vi "PM100D_Initialize.vi"() -> (4 "VISA out":refnum<visa-resource-name>, 6 "Ranges":string[](array[string]), 8 "Instrument":string, 10 "Connected":bool, 15 "error out":errorcluster)   [LabVIEW 2015]
doc: "This VI scans for connected devices, that can be selected in a dialog box. Next steps\n- setting timeout\n- performing identification query\n- configuring the operation register to '512'; flag gets to HI when a new measurement value is ready to fetch\n- clear operation register"
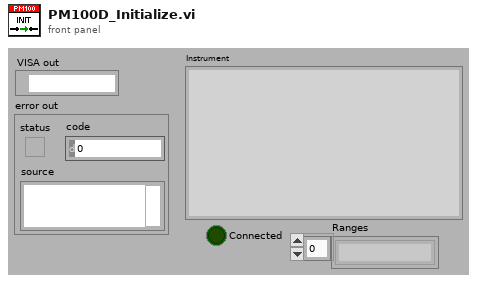
[diagram p1: front panel]
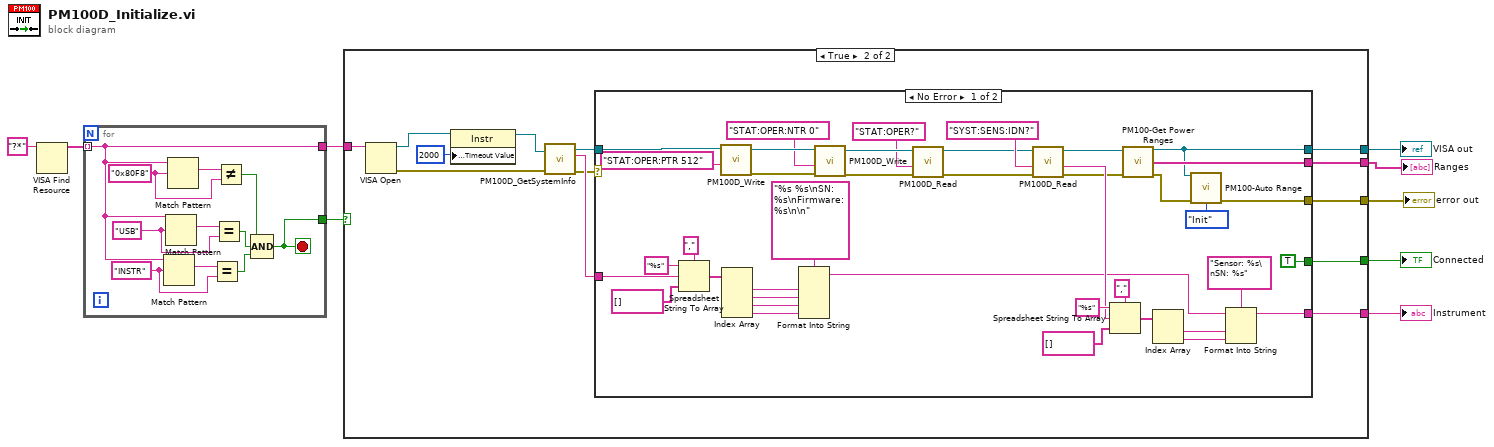
[diagram p0: block diagram]
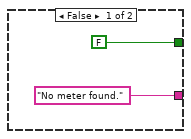
[diagram p2: hidden frame]
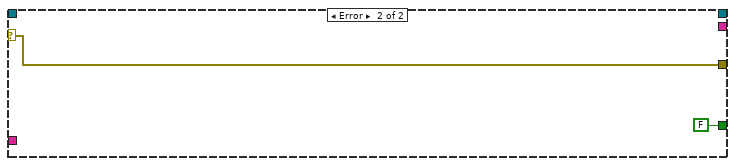
[diagram p3: hidden frame]
diagram:
  n1 = VISA Find Resource(11:"?*" ("expression (\"?*\")")) -> (3:w6:string[])  [unwired: 1 in, 3 out]
  n2 = for {
    tunnel: w6 -> [w11] mode=indexing
    tunnel: [w11] -> w5
    tunnel: [w10] -> w4
    stop <- w10 stop-if-true
    w12 = "0x80F8" ("regular expression")
    w18 = "INSTR" ("regular expression")
    w16 = "USB" ("regular expression")
    n3 = Match Pattern(string=w11, regular expression=w18) -> (match substring=w17:string)  [unwired: 1 in, 3 out]
    n4 = Match Pattern(string=w11, regular expression=w16) -> (match substring=w15:string)  [unwired: 1 in, 3 out]
    n5 = Match Pattern(string=w11, regular expression=w12) -> (match substring=w14:string)  [unwired: 1 in, 3 out]
    n6 = Equal?(x=w17, y=w18) -> (x = y?=w20:bool)
    n7 = Equal?(x=w15, y=w16) -> (x = y?=w19:bool)
    n8 = Not Equal?(x=w14, y=w12) -> (x != y?=w13:bool)
    n9 = Compound Arithmetic op=AND(w13, w19, w20) -> (w10:bool)
  }
  n10 = case shown="True" w4 {
    tunnel: [_ w25] -> w2
    tunnel: [_ w24] -> w9
    tunnel: ["No meter found." w28] -> w8
    tunnel: w5 -> [_ w27]
    tunnel: [FALSE w26] -> w3
    tunnel: [_ w23] -> w1
    frame False {
    }
    frame True {
      n11 = VISA Open(VISA resource name=w27) -> (VISA resource name=w33:refnum<visa-resource-name>, error out=w35:errorcluster)  [unwired: 1 in, 3 out]
      n12 = property class="Instr"(reference=w33, "General Settings:Timeout Value"=u32 2000) -> (reference out=w32:refnum<visa-resource-name>)  [unwired: 1 in, 1 out]
      n13 = call "PM100D_GetSystemInfo.vi"("VISA in"=w32, "error in"=w35) -> ("VISA out"=w31:refnum<visa-resource-name>, "Instrument"=w30:string, "error out"=w29:errorcluster)  [unwired: 1 out]
      n14 = case shown="No Error" w29 {
        selector: w29 -> [_ w76]
        tunnel: w31 -> [w73 _]
        tunnel: [w40 _] -> w25
        tunnel: [w38 w76] -> w24
        tunnel: w30 -> [w64 _]
        tunnel: [w48 _] -> w28
        tunnel: [TRUE FALSE] -> w26
        tunnel: [w43 _] -> w23
        frame No Error {
          n15 = Spreadsheet String To Array(delimiter (Tab)=",", format string="%s", spreadsheet string=w64, array type (2D Dbl)=string[] [] ("Rng_Array")) -> (array=w57:string[])
          n16 = call "PM100D_Write.vi"("Command"="STAT:OPER:PTR 512", "VISA in"=w73) -> ("error out"=w71:errorcluster, "VISA out"=w72:refnum<visa-resource-name>)  [unwired: 8 in]
          n17 = Index Array(array=w57) -> (element #1=w61:string, element #2=w60:string, element #3=w59:string, element #4=w58:string)  [unwired: 4 in]
          n18 = Format Into String(format string="%s %s\nSN: %s\nFirmware: %s\n\n", w61, w60, w59, w58) -> (resulting string=w47:string)  [unwired: 2 in, 1 out]
          n19 = call "PM100D_Write.vi"("error in (no error)"=w71, "Command"="STAT:OPER:NTR 0", "VISA in"=w72) -> ("error out"=w67:errorcluster, "VISA out"=w69:refnum<visa-resource-name>)  [unwired: 7 in]
          n20 = call "PM100D_Read.vi"("error in (no error)"=w67, "Command"="STAT:OPER?", "VISA in"=w69) -> ("error out"=w56:errorcluster, "VISA out"=w36:refnum<visa-resource-name>)  [unwired: 6 in, 1 out]
          n21 = call "PM100D_Read.vi"("error in (no error)"=w56, "Command"="SYST:SENS:IDN?", "VISA in"=w36) -> ("error out"=w41:errorcluster, "ReadValue"=w50:string, "VISA out"=w42:refnum<visa-resource-name>)  [unwired: 6 in]
          n22 = Spreadsheet String To Array(delimiter (Tab)=",", format string="%s", spreadsheet string=w50, array type (2D Dbl)=string[] [] ("Rng_Array")) -> (array=w51:string[])
          n23 = call "PM100-Get Power Ranges.vi"("VISA Refnum in"=w42, "error in (no error)"=w41) -> ("VISA Refnum out"=w40:refnum<visa-resource-name>, "Ranges"=w43:string[], "error out"=w39:errorcluster)  [unwired: 11 in]
          n24 = Index Array(array=w51) -> (element #1=w46:string, element #2=w45:string)  [unwired: 2 in]
          n25 = call "PM100-Auto Range.vi"("VISA in"=w40, "error in (no error)"=w39, "Action"=enum16{"Init", "Apply"}."Init") -> ("error out"=w38:errorcluster)  [unwired: 12 in]
          n26 = Format Into String(format string="Sensor: %s\nSN: %s", initial string=w47, w46, w45) -> (resulting string=w48:string)  [unwired: 1 in, 1 out]
        }
        frame Error {
        }
      }
    }
  }
  "VISA out" <- w2
  "error out" <- w9
  "Instrument" <- w8
  "Connected" <- w3
  "Ranges" <- w1
